vi "Car Simulation-demo.vi"() -> ()   [LabVIEW 2020]
uses:
  <vilib>/event_ctls.llb/eventvkey.ctl
  <vilib>/numeric/Random Number (Range) I64.vi
  <vilib>/numeric/sub_Random U32.vi
panel:
  out "realdir":dbl format="%#_3g"
  in  "show mistake":bool
  in  "no road/road?":bool=TRUE
  out "velocity":cluster{"x":dbl, "y":dbl}
  in  "VKey 2":T1=enum."Ctrl"
  in  "Backward?":bool
  out "String":string
  out "location":T2
  out "readings":T3
  out "buffer":T4
  in  "y buffer":dbl
  in  "x buffer":dbl
  in  "end game":bool
  in  "Brake Pin":i32=2
  in  "Accelerator Pin":i32=1
  in  "xAccelerometer Pin":i32
  in  "Road Width":i8=7 min=5 max=11 step=2
  in  "Pause/Start":bool
  out "map":bool[][](array[boolean])
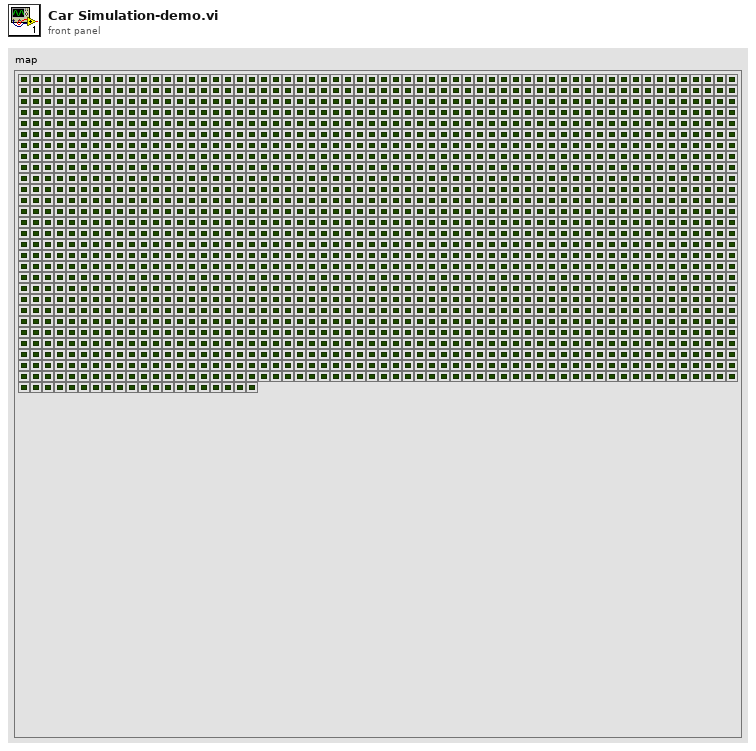
[diagram p1: front panel]
types:
  T1 = typedef "eventvkey.ctl" = enum16{"ASCII", "Enter", "Return", "Shift", "Ctrl", "Alt", "Cmd", "Opt", "Caps", "NumLock", "Clear", "Break", "Up", "Down", "Left", "Right", "Insert", "Delete", "Home", "End", "PageUp", "PageDown", "Escape", "Help", "Pause", "ScrollLock", "F1", "F2", "F3", "F4", "F5", "F6", "F7", "F8", "F9", "F10", "F11", "F12", "F13", "F14", "F15", "F16", "F17", "F18", "F19", "F20", "F21", "F22", "F23", "F24", "Play", "VolumeUp", "VolumeDown", "Mute", "Two Byte Char"}
  T2 = cluster{"Row":i64, "Column":i64, "Direction":i64}
  T3 = cluster{"xAccelerometer":dbl, "accelerator":dbl, "brake":dbl}
  T4 = cluster{"x buffer":dbl, "y buffer":dbl, "real direction":dbl}
  T5 = cluster{"number":i64, "number":i64, "number":i64}
  T6 = cluster{"Handle":i32, "xAccelerometer Pin":i32, "Accelerator Pin":i32, "Brake Pin":i32}
  T7 = cluster{"Row":i32, "Column":i32, "Direction":i32}
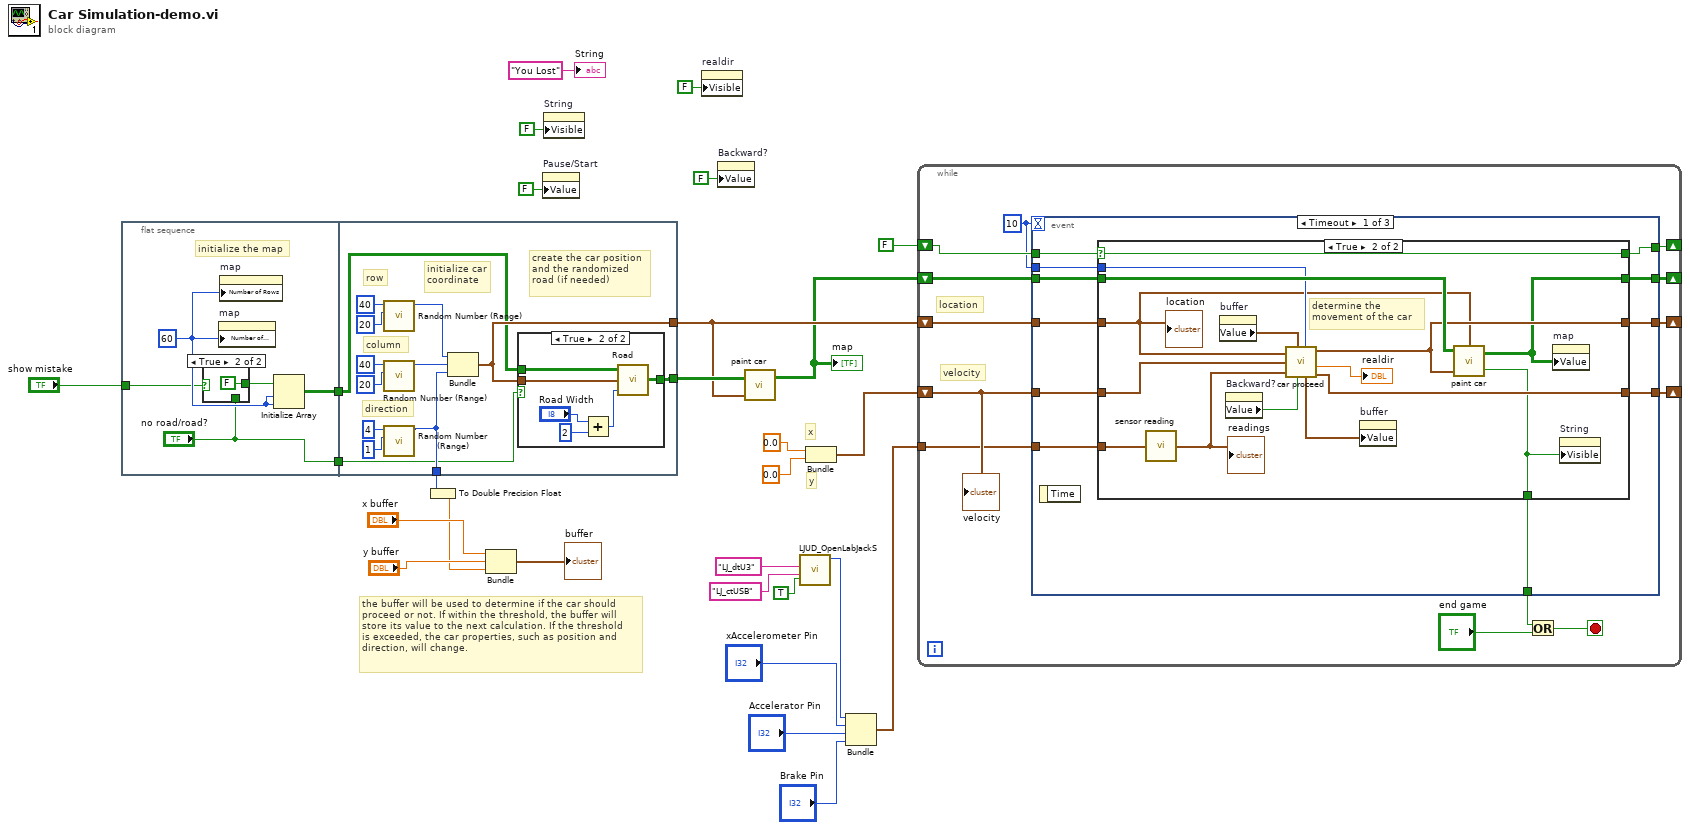
[diagram p0: block diagram]
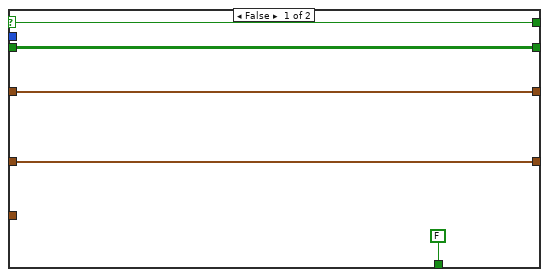
[diagram p2: hidden frame]
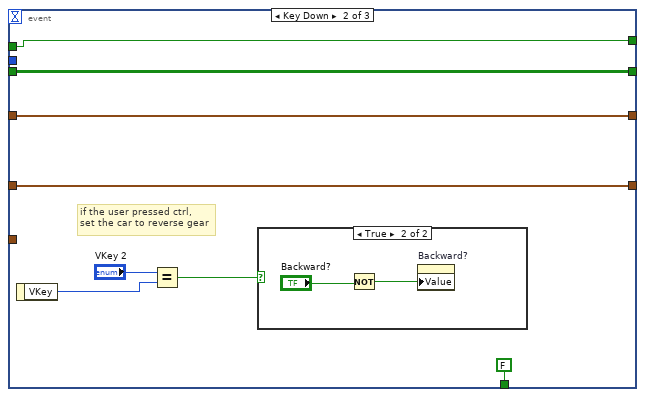
[diagram p3: hidden frame]
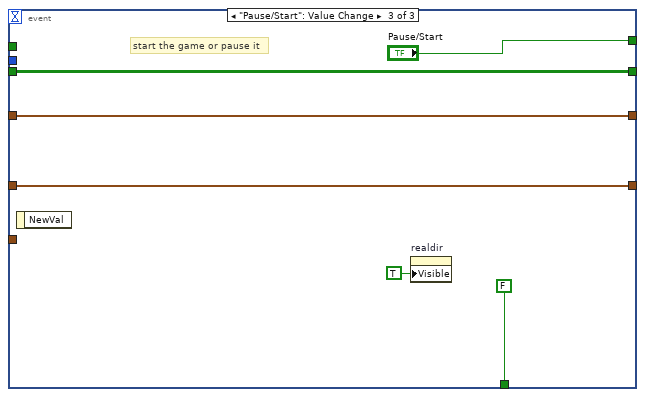
[diagram p5: hidden frame]
diagram:
  # "the buffer will be used to determine if the car should\nproceed or not. If within the threshold, the buffer will\nstore its value to the next calculation. If the threshold\nis exceeded, the car properties, such as position and\ndirection, will change."
  # "y"
  # "x"
  n1 = flat-sequence {
    tunnel: [w33] -> w27
    tunnel: ["no road/road?"] -> w10
    tunnel: "show mistake" -> [w30]
    tunnel: [w41] -> w25
    tunnel: w27 -> [w40]
    tunnel: [w44] -> w26
    tunnel: [w39] -> w12
    tunnel: w10 -> [w36]
    frame #0 {
      w32 = u32 60 ("Number of Columns")
      # "initialize the map"
      n2 = case shown="True" w30 {
        tunnel: [w34 FALSE ("element")] -> w31
        tunnel: "no road/road?" -> [w34 _]
        frame False {
        }
        frame True {
        }
      }
      n3 = property on="map" class="Arr (strict)"("Number of Columns"=w32) -> ()  [unwired: 2 in, 2 out]
      n4 = property on="map" class="Arr (strict)"("Number of Rows"=w32) -> ()  [unwired: 2 in, 2 out]
      n5 = Initialize Array(w31, w32, w32) -> (w33:bool[][])
    }
    frame #1 {
      # "initialize car\ncoordinate"
      # "create the car position\nand the randomized\nroad (if needed)"
      # "direction"
      # "column"
      # "row"
      n6 = call-poly <vilib>:"Random Number (Range).vi"("lower bound (-100)"=i64 20, "upper bound (100)"=i64 40) -> ("number"=w43:i64)  [unwired: 9 in]
      n7 = call-poly <vilib>:"Random Number (Range).vi"("lower bound (-100)"=i64 20, "upper bound (100)"=i64 40) -> ("number"=w42:i64)  [unwired: 9 in]
      n8 = call-poly <vilib>:"Random Number (Range).vi"("lower bound (-100)"=i64 1, "upper bound (100)"=i64 4) -> ("number"=w39:i64)  [unwired: 9 in]
      n9 = Bundle("number"=w43, "number"=w42, "number"=w39) -> (w41:T5)  [unwired: 1 in]
      n10 = case shown="True" w36 {
        tunnel: [w49 w55] -> w44
        tunnel: w41 -> [_ w51]
        tunnel: w40 -> [w49 w50]
        frame False {
        }
        frame True {
          n11 = Add(x="Road Width", y=i8 2) -> (x+y=w52:i8)
          n12 = call "Road.vi"("Road Width"=w52, "coordinate"=w51, "Map in"=w50) -> ("Map out"=w55:bool[][])
        }
      }
    }
  }
  n13 = To Double Precision Float(number=w12) -> (double precision float=w11:dbl)
  n14 = Bundle("x buffer"="x buffer", "y buffer"="y buffer", w11) -> (→"buffer":cluster{"x buffer":dbl, "y buffer":dbl, dbl})  [unwired: 1 in]
  n15 = property on="Pause/Start" class="Bool (strict)"("Value"=FALSE ("Start/Stop")) -> ()  [unwired: 2 in, 2 out]
  n16 = property on="String" class="Str"("Visible"=FALSE) -> ()  [unwired: 2 in, 2 out]
  n17 = property on="realdir" class="DigNum (strict)"("Visible"=FALSE) -> ()  [unwired: 2 in, 2 out]
  n18 = property on="Backward?" class="Bool (strict)"("Value"=FALSE ("Backward?")) -> ()  [unwired: 2 in, 2 out]
  n19 = call "paint car.vi"("New Location"=w25, "Map in"=w26) -> ("Map out"=w16:bool[][])  [unwired: 2 in, 1 out]
  "map" <- w16
  n20 = call <vilib>:"LJUD_OpenLabJackS.vi"("FirstFound"=TRUE, "ConnectionType"="LJ_ctUSB", "DeviceType"="LJ_dtU3") -> ("Handle"=w2:i32)  [unwired: 6 in, 2 out]
  n21 = Bundle("element"=0.0, "element"=0.0) -> (w21:cluster{"element":dbl, "element":dbl})  [unwired: 1 in]
  n22 = Bundle("Handle"=w2, "xAccelerometer Pin"="xAccelerometer Pin", "Accelerator Pin"="Accelerator Pin", "Brake Pin"="Brake Pin") -> (w24:T6)  [unwired: 1 in]
  n23 = while {
    shift-right: [w68] -> _
    shift-left: FALSE ("Start/Stop") -> [w67]
    shift-right: [w63] -> _
    shift-left: w25 -> [w66]
    shift-right: [w62] -> _
    shift-left: w21 -> [w65]
    tunnel: w24 -> [w64]
    shift-right: [w59] -> _
    shift-left: w16 -> [w60]
    stop <- w57 stop-if-true
    w61 = 10
    # "velocity"
    # "location"
    n24 = event shown="[0] Timeout" {
      selector: _ -> [_ _ _]
      dyn-events: _ -> [_ _ _]
      timeout: w61 -> [_ _ _]
      tunnel: [w78 w107 "Pause/Start"] -> w68
      tunnel: w67 -> [w79 w107 _]
      tunnel: w66 -> [w77 w105 w113]
      tunnel: w65 -> [w76 w104 w112]
      tunnel: w64 -> [w75 _ _]
      tunnel: [w74 w105 w113] -> w63
      tunnel: [w73 w104 w112] -> w62
      tunnel: w61 -> [w72 _ _]
      tunnel: w60 -> [w71 w106 w114]
      tunnel: [w70 w106 w114] -> w59
      tunnel: [w69 FALSE ("hit?") FALSE ("hit?")] -> w56
      event Timeout {
        n25 = event-data() -> ()  [unwired: 1 in, 1 out]
        n26 = case shown="True" w79 {
          selector: w79 -> [w84 w99]
          tunnel: [w84 w99] -> w78
          tunnel: w77 -> [w83 w88]
          tunnel: w76 -> [w82 w97]
          tunnel: w75 -> [_ w98]
          tunnel: [w83 w92] -> w74
          tunnel: [w82 w94] -> w73
          tunnel: w72 -> [_ w89]
          tunnel: w71 -> [w81 w93]
          tunnel: [w81 w91] -> w70
          tunnel: [FALSE ("hit?") w90] -> w69
          frame False {
          }
          frame True {
            # "determine the\nmovement of the car"
            n27 = call "sensor reading.vi"("Input parameter"=w98) -> ("readings"=w96:T3)
            "readings" <- w96
            n28 = property on="buffer" class="Clust (strict)"() -> ("Value"=w95:T4)  [unwired: 2 in, 2 out]
            n29 = property on="Backward?" class="Bool (strict)"() -> ("Value"=w86:bool)  [unwired: 2 in, 2 out]
            n30 = call "car proceed.vi"("location in"=w88, "old buffer"=w95, "velocity in"=w97, "sensor reading"=w96, "Backward?"=w86, "refresh rate"=w89) -> ("location out"=w92:T7, "new buffer"=w87:T4, "realdir"=→"realdir":dbl, "velocity out"=w94:cluster{"x":dbl, "y":dbl})  [unwired: 1 in]
            n31 = property on="buffer" class="Clust (strict)"("Value"=w87) -> ()  [unwired: 2 in, 2 out]
            n32 = call "paint car.vi"("Old Location"=w88, "New Location"=w92, "Map in"=w93) -> ("hit?"=w90:bool, "Map out"=w91:bool[][])  [unwired: 1 in]
            n33 = property on="map" class="Arr (strict)"("Value"=w91) -> ()  [unwired: 2 in, 2 out]
            n34 = property on="String" class="Str"("Visible"=w90) -> ()  [unwired: 2 in, 2 out]
            "location" <- w88
          }
        }
      }
      event Key Down {
        # "if the user pressed ctrl,\nset the car to reverse gear"
        n35 = event-data() -> ("VKey"=w101:T1)  [unwired: 1 in]
        n36 = Equal?(x="VKey 2", y=w101) -> (x = y?=w100:bool)
        n37 = case shown="True" w100 {
          frame False {
          }
          frame True {
            n38 = Not(x="Backward?") -> (.not. x?=w108:bool)
            n39 = property on="Backward?" class="Bool (strict)"("Value"=w108) -> ()  [unwired: 2 in, 2 out]
          }
        }
      }
      event "Pause/Start": Value Change {
        # "start the game or pause it"
        n40 = event-data() -> ()  [unwired: 1 in, 1 out]
        n41 = property on="realdir" class="DigNum (strict)"("Visible"=TRUE) -> ()  [unwired: 2 in, 2 out]
      }
    }
    n42 = Or(x=w56, y="end game") -> (x .or. y?=w57:bool)
    "velocity" <- w65
  }
  "String" <- "You Lost" ("String")
